vi "FTW-CodeGen-Prototype.vi"(0 "REPLACED_Data Type and Default Values":variant, 5 "REPLACED_JSON String":string, 11 "REPLACED_error in":errorcluster) -> (4 "REPLACED_Populated Values":variant, 15 "REPLACED_error out":errorcluster)   [LabVIEW 2012, in "FTW-JSON-Deserialize.xnode"]
uses:
  FTW-JSON-Deserialize.xnode
  src/Regex/FTW-Regex.vi
  src/JSON/FTW-JSON-RegexHeader.vi
  src/Error/FTW-ERR-ThrowError.vi
  src/Container/FTW-Container.lvclass
panel:
  # "Inputs"
  # "Outputs"
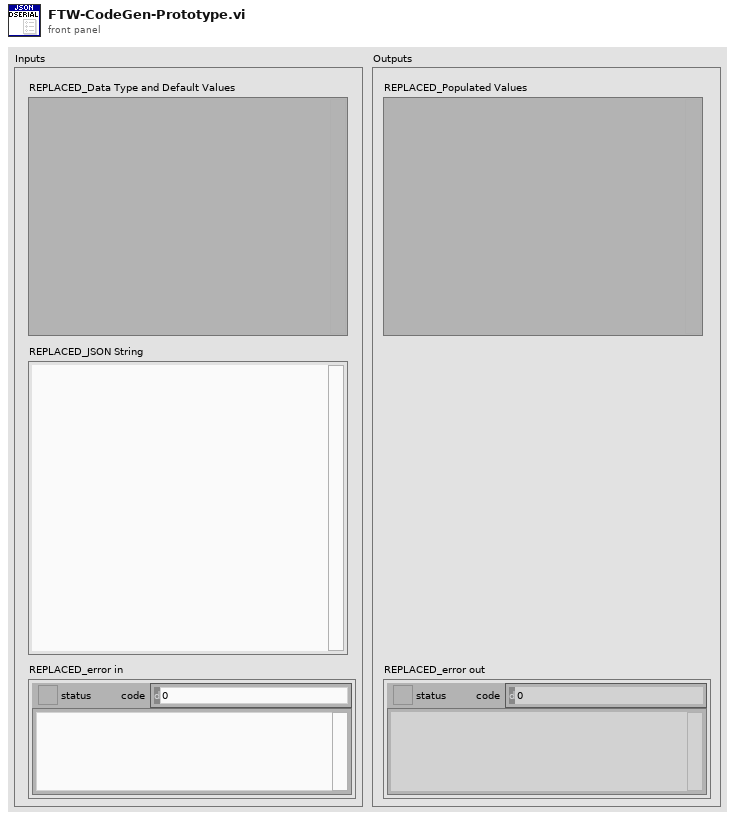
[diagram p1: front panel]
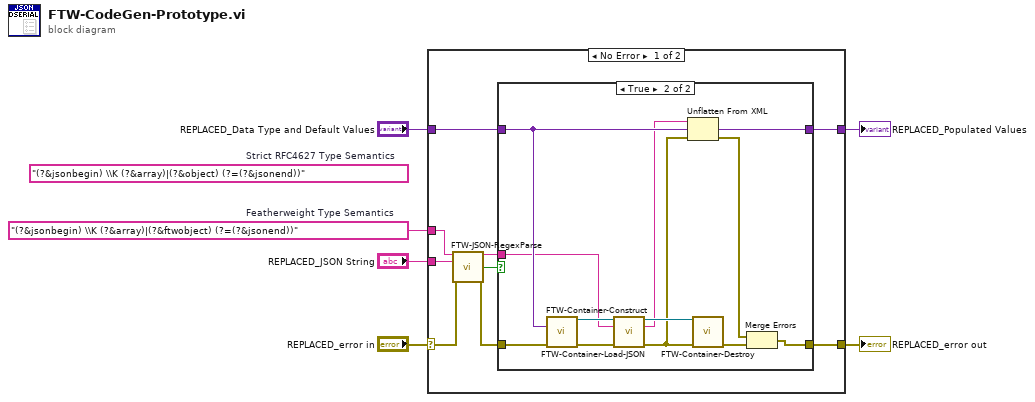
[diagram p0: block diagram]
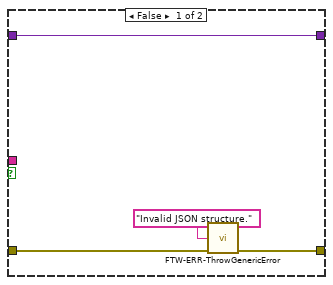
[diagram p2: hidden frame]
diagram:
  (unwired) "(?&jsonbegin) \\K (?&array)|(?&object) (?=(?&jsonend))"  # Strict RFC4627 Type Semantics
  w1 = "(?&jsonbegin) \\K (?&array)|(?&ftwobject) (?=(?&jsonend))"  # Featherweight Type Semantics
  n1 = case shown="No Error" "REPLACED_error in" {
    selector: "REPLACED_error in" -> [w9 w32]
    tunnel: "REPLACED_JSON String" -> [w15 _]
    tunnel: "REPLACED_Data Type and Default Values" -> [w14 w33]
    tunnel: [w13 w33] -> w4
    tunnel: [w10 w32] -> w3
    tunnel: w1 -> [w7 _]
    frame No Error {
      n2 = call "FTW-JSON-RegexParse.vi"("Regular Expression using JSON subroutines"=w7, "Input String"=w15, "error in"=w9) -> ("Match"=w12:string, "Found Match?"=w8:bool, "error out"=w11:errorcluster)  [unwired: 8 in, 2 out]
      n3 = case shown="True" w8 {
        tunnel: w14 -> [w16 w28]
        tunnel: [w16 w31] -> w13
        tunnel: w12 -> [_ w25]
        tunnel: w11 -> [w19 w27]
        tunnel: [w18 w29] -> w10
        frame False {
          n4 = call "FTW-ERR-ThrowGenericError.vi"("Error Message"="Invalid JSON structure.", "error in"=w19) -> ("error out"=w18:errorcluster)  [unwired: 13 in]
        }
        frame True {
          n5 = call "FTW-Container-Construct.vi"("LabVIEW Data Structure"=w28, "error in"=w27) -> ("Container"=w26:refnum<class "FTW-Container.lvclass">, "error out"=w23:errorcluster)  [unwired: 12 in]
          n6 = call "FTW-Container-Load-JSON.vi"("Container"=w26, "JSON to Load"=w25, "error in"=w23) -> ("Container out"=w24:refnum<class "FTW-Container.lvclass">, "Serialized Node"=w20:string, "error out"=w21:errorcluster)  [unwired: 10 in]
          n7 = Unflatten From XML(xml string=w20, type=w28, error in (no error)=w21) -> (value=w31:variant, error out=w30:errorcluster)
          n8 = call "FTW-Container-Destroy.vi"("Container"=w24, "error in"=w21) -> ("error out"=w22:errorcluster)  [unwired: 13 in]
          n9 = Merge Errors(w30, w22) -> (w29:errorcluster)
        }
      }
    }
    frame Error {
    }
  }
  "REPLACED_error out" <- w3
  "REPLACED_Populated Values" <- w4
